vi "FormaCanonicaControlable.vi"(0 "Num":dbl[](array[numeric]), 1 "Den":dbl[](array[numeric]), 2 "Xi":T1, 3 "Retardo padé":dbl, 4 "dt":dbl, 5 "u(k)":dbl) -> (14 "Num":string, 15 "Den":string, 16 "String Retardo":string, 17 "x(k)":T1, 18 "y(k)":dbl)   [LabVIEW 2019]
uses:
  <vilib>/Analysis/Matrix/Datatypes/RealMatrix.ctl
  <vilib>/Analysis/baseanly.llb/Real A x B.vi
  <vilib>/Analysis/Matrix/Numeric/Conversions/Array To Matrix - RA.vi
  <vilib>/Analysis/Matrix/Numeric/Add/Add - RM,RM.vi
  <vilib>/Analysis/Matrix/Numeric/Multiply/Multiply - RM,R.vi
  <vilib>/Analysis/Matrix/Numeric/Conversions/Array To Matrix - RA2.vi
  <vilib>/Analysis/Matrix/Comparison/Equal/Equal - RM,RM.vi
  <vilib>/Analysis/Matrix/Numeric/Multiply/Multiply - R,RM.vi
  <vilib>/Analysis/Matrix/NI_Matrix.lvlib
  <vilib>/Analysis/NI_AALBase.lvlib
panel:
  # "B"
  # "A"
  # "C"
  # "D"
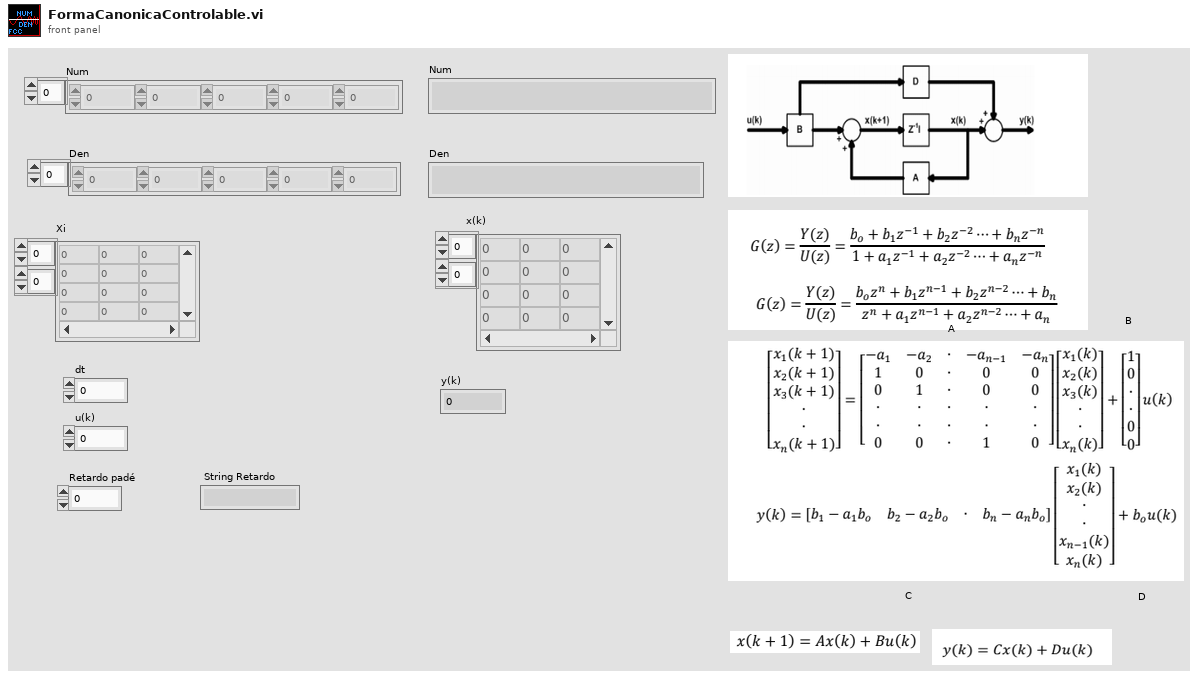
[diagram p1: front panel]
types:
  T1 = typedef "NI_Matrix.lvlib/RealMatrix.ctl" = dbl[][]
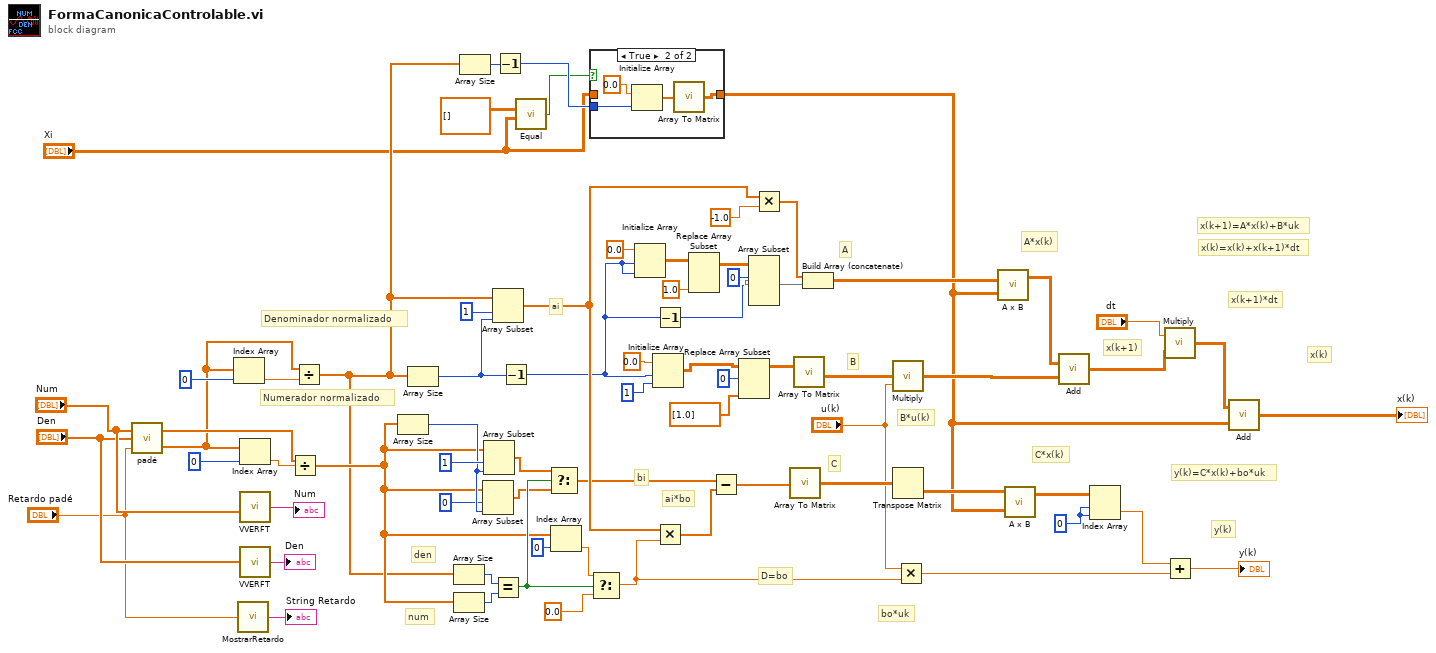
[diagram p0: block diagram]
diagram:
  w23 = 0 ("index (row)")
  # "bi"
  # "ai"
  # "Numerador normalizado"
  # "num"
  # "den"
  # "bo*uk"
  # "y(k)"
  # "y(k)=C*x(k)+bo*uk"
  # "x(k+1)=A*x(k)+B*uk"
  # "x(k)"
  # "x(k)=x(k)+x(k+1)*dt"
  # "C*x(k)"
  # "x(k+1)*dt"
  # "x(k+1)"
  # "B*u(k)"
  # "A*x(k)"
  # "ai*bo"
  # "D=bo"
  # "C"
  # "B"
  # "A"
  # "Denominador normalizado"
  n1 = call "padé.vi"("Retardo padé"="Retardo padé", "Den"="Den", "Num"="Num") -> ("DEN"=w13:dbl[], "NUM"=w14:dbl[])
  n2 = Index Array(array=w13, index=0) -> (element=w64:dbl)
  n3 = call "MostrarRetardo.vi"("Retardo"="Retardo padé") -> ("String Retardo"=→"String Retardo":string)
  n4 = Index Array(array=w13, index=0) -> (element=w17:dbl)
  n5 = call "VVERFT.vi"("Vector"="Num") -> ("Funcion de transferencia"=→"Num":string)
  n6 = call "VVERFT.vi"("Vector"="Den") -> ("Funcion de transferencia"=→"Den":string)
  n7 = Divide(x=w14, y=w17) -> (x/y=w16:dbl[])
  n8 = Divide(x=w13, y=w64) -> (x/y=w9:dbl[])
  n9 = Array Size(array=w16) -> (size(s)=w34:i32)
  n10 = Array Size(array=w9) -> (size(s)=w15:i32)
  n11 = Array Size(array=w9) -> (size(s)=w42:i32)
  n12 = Array Size(array=w16) -> (size(s)=w41:i32)
  n13 = Array Size(array=w9) -> (size(s)=w8:i32)
  n14 = Array Subset(array=w16, index=0, length=w34) -> (w32:dbl[])
  n15 = Array Subset(array=w16, index=1, length=w34) -> (w36:dbl[])
  n16 = Array Subset(array=w9, index=1, length=w15) -> (w50:dbl[])
  n17 = Equal?(x=w42, y=w41) -> (x = y?=w37:bool)
  n18 = Decrement(x=w8) -> (x-1=w7:i32)
  n19 = Decrement(x=w15) -> (x-1=w48:i32)
  n20 = call-poly <vilib>:"Equal.vi"("Real Matrix B"="Xi", "Real Matrix A"=T1 [] ("x(k)")) -> ("A = B?"=w5:bool)
  n21 = Select(t=w36, s=w37, f=w32) -> (s? t:f=w31:dbl[])
  n22 = Index Array(array=w16, index=0) -> (element=w40:dbl)
  n23 = case shown="True" w5 {
    tunnel: w7 -> [_ w75]
    tunnel: [w71 w72] -> w3
    tunnel: "Xi" -> [w71 _]
    frame False {
    }
    frame True {
      n24 = Initialize Array(0.0 ("element"), w75) -> (w73:dbl[])
      n25 = call-poly <vilib>:"Array To Matrix.vi"("Real 1D Array"=w73) -> ("Real Matrix (Column Vector)"=w72:T1)
    }
  }
  n26 = Select(t=w40, s=w37, f=0.0) -> (s? t:f=w30:dbl)
  n27 = Initialize Array(0.0 ("element"), w48, w48) -> (w70:dbl[][])
  n28 = Initialize Array(0.0 ("element"), w48, 1 ("dimension size")) -> (w57:dbl[][])
  n29 = Decrement(x=w48) -> (x-1=w49:i32)
  n30 = Multiply(x=w50, y=w30) -> (x*y=w53:dbl[])
  n31 = Replace Array Subset(array=w70, new element=1.0 ("new diagonal/fill element")) -> (w67:T1)  [unwired: 2 in]
  n32 = Subtract(x=w31, y=w53) -> (x-y=w38:dbl[])
  n33 = Replace Array Subset(array=w57, new element=dbl[] [1.0] ("new element/subarray"), index (row)=0 ("index")) -> (w55:dbl[][])  [unwired: 1 in]
  n34 = Array Subset(array=w67, index (row)=0 ("index"), length (row)=w49) -> (w65:T1)  [unwired: 2 in]
  n35 = Multiply(x=w50, y=-1.0) -> (x*y=w52:dbl[])
  n36 = call-poly <vilib>:"Array To Matrix.vi"("Real 1D Array"=w38) -> ("Real Matrix (Column Vector)"=w51:T1)
  n37 = call-poly <vilib>:"Array To Matrix.vi"("Real 2D Array"=w55) -> ("Real Matrix"=w19:T1)
  n38 = Build Array (concatenate)(w52, w65) -> (w47:T1)
  n39 = call-poly <vilib>:"Multiply.vi"("Real Scalar c"="u(k)", "Real Matrix A"=w19) -> ("A * c"=w27:T1)
  n40 = Transpose Matrix(1:w51) -> (0:w46:T1)
  n41 = Multiply(x="u(k)", y=w30) -> (x*y=w21:dbl)
  n42 = call-poly <vilib>:"A x B.vi"("B"=w3, "A"=w47) -> ("A x B"=w28:T1)  [unwired: 1 out]
  n43 = call-poly <vilib>:"A x B.vi"("B"=w3, "A"=w46) -> ("A x B"=w24:T1)  [unwired: 1 out]
  n44 = call-poly <vilib>:"Add.vi"("Real Matrix B"=w27, "Real Matrix A"=w28) -> ("A + B"=w26:T1)
  n45 = Index Array(array=w24, index (row)=w23, index (col)=w23) -> (element=w22:dbl)
  n46 = call-poly <vilib>:"Multiply.vi"("Real Matrix A"=w26, "Real Scalar c"="dt") -> ("c * A"=w25:T1)
  n47 = Add(x=w22, y=w21) -> (x+y=→"y(k)":dbl)
  n48 = call-poly <vilib>:"Add.vi"("Real Matrix B"=w3, "Real Matrix A"=w25) -> ("A + B"=→"x(k)":T1)
